vi "Get Data Marker Name [DM].vi"(8 "error in (no error)":errorcluster, 9 "Name Buffer Size":i32 format="%.0g", 10 "Marker Index (1)":i32=1 format="%.0g", 11 "CS++Fgen in":refnum<class "CS++Fgen.lvclass">) -> (0 "error out":errorcluster, 2 "Marker Name":string, 3 "CS++Fgen out":refnum<class "CS++Fgen.lvclass">)   [LabVIEW 2013, in "CS++Fgen.lvlib" / "CS++Fgen.lvclass"]
doc: "This VI returns the repeated capability identifier for the data marker that corresponds to the one-based index you specify. If the value that you pass for the Index control is less than one or greater than the value of the data marker count, the VI returns an empty string in the Name control and returns an error.\n\nNote:\n\n(1) This VI is part of the IviFgenDataMarker [DM] extension group."
uses:
  CS++Fgen.lvclass
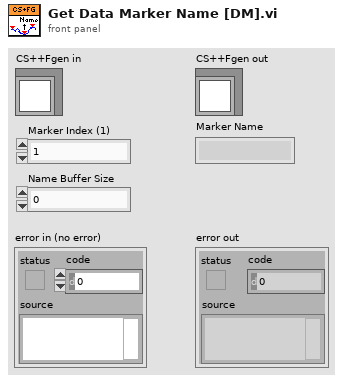
[diagram p1: front panel]
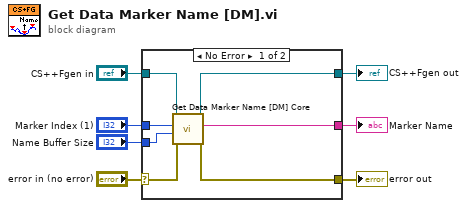
[diagram p0: block diagram]
diagram:
  n1 = case shown="No Error" "error in (no error)" {
    selector: "error in (no error)" -> [w11 w16]
    tunnel: [w12 w16] -> w6
    tunnel: [w13 w15] -> w4
    tunnel: "CS++Fgen in" -> [w14 w15]
    tunnel: "Marker Index (1)" -> [w10 _]
    tunnel: "Name Buffer Size" -> [w9 _]
    tunnel: [w8 _] -> w1
    frame No Error {
      n2 = call-dynamic "Get Data Marker Name [DM] Core.vi"("error in (no error)"=w11, "Name Buffer Size"=w9, "Marker Index (1)"=w10, "CS++Fgen in"=w14) -> ("error out"=w12:errorcluster, "Marker Name"=w8:string, "CS++Fgen out"=w13:refnum<class "CS++Fgen.lvclass">)  [unwired: 5 in]
    }
    frame Error {
    }
  }
  "error out" <- w6
  "CS++Fgen out" <- w4
  "Marker Name" <- w1
